vi "Read Labels Temperatures.vi"(11 "Slave ID":dbl) -> (3 "Etykiety T1-10":T1)   [LabVIEW 2017]
uses:
  <vilib>/Utility/config.llb/NI_LVConfig.lvlib
panel:
  in  "Etykiety T1-10":T1
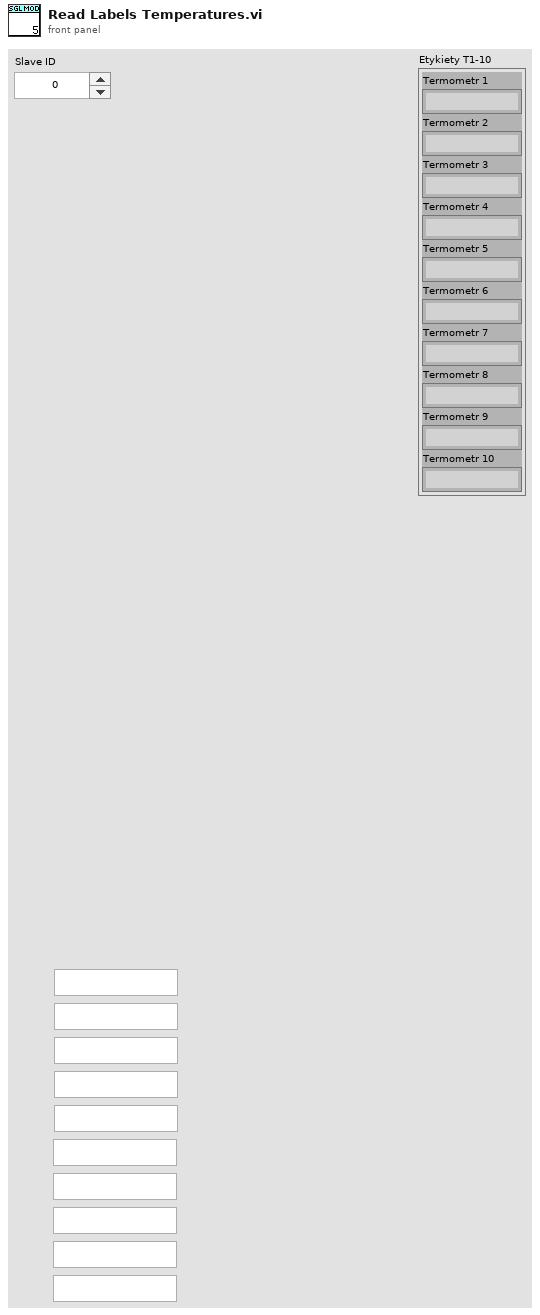
[diagram p1: front panel]
types:
  T1 = cluster{"Termometr 1":string, "Termometr 2":string, "Termometr 3":string, "Termometr 4":string, "Termometr 5":string, "Termometr 6":string, "Termometr 7":string, "Termometr 8":string, "Termometr 9":string, "Termometr 10":string}
  T2 = typedef "NI_LVConfig.lvlib/Config Data RefNum.ctl" = refnum<k1>
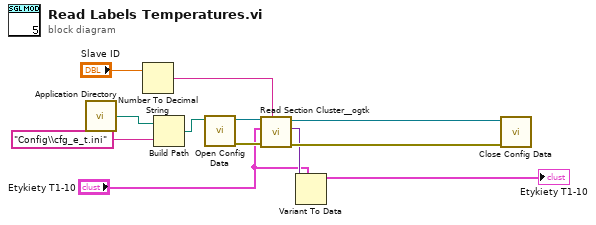
[diagram p0: block diagram]
diagram:
  n1 = call <vilib>:"Application Directory.vi"() -> ("Application Directory"=w8:path)
  n2 = Number To Decimal String(number="Slave ID") -> (decimal integer string=w10:string)  [unwired: 1 in]
  n3 = Build Path(base path=w8, name or relative path="Config\\cfg_e_t.ini") -> (appended path=w6:path)
  n4 = call <vilib>:"Open Config Data.vi"("configuration file path"=w6) -> ("error out"=w5:errorcluster, "refnum"=w4:T2)  [unwired: 8 in, 1 out]
  n5 = call <userlib>:"Read Section Cluster__ogtk.vi"("section (optional)"=w10, "error in (no error)"=w5, "Section Formatted Cluster Type"="Etykiety T1-10", "refnum"=w4) -> ("error out"=w12:errorcluster, "Section Formatted Cluster"=w9:variant, "dup refnum"=w11:T2)  [unwired: 3 in, 2 out]
  n6 = Variant To Data(type="Etykiety T1-10", Variant=w9) -> (data=→"Etykiety T1-10":T1)  [unwired: 1 in, 1 out]
  n7 = call <vilib>:"Close Config Data.vi"("error in (no error)"=w12, "refnum"=w11) -> ()  [unwired: 8 in, 2 out]
